vi "ReadSeq_Analyze.vi"(6 "RotateAngle":string, 7 "Color":u32(colorbox)=16711680, 8 "error in (no error)":errorcluster, 9 "Cam Index":i32, 10 "script path":string, 11 "coordinate space":bool) -> (0 "error out":errorcluster, 1 "data string":string, 2 "Description":string, 3 "VarName":string)   [LabVIEW 2015]
panel:
  out "x-y":u32
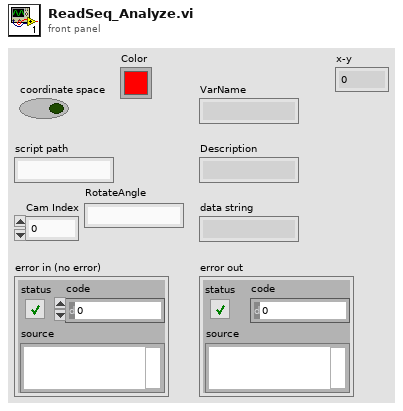
[diagram p1: front panel]
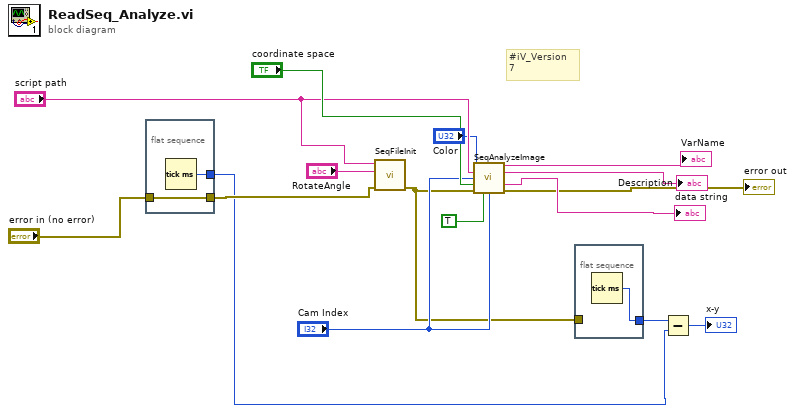
[diagram p0: block diagram]
diagram:
  # "#iV_Version\n7"
  n1 = flat-sequence {
    tunnel: "error in (no error)" -> [w18]
    tunnel: [w18] -> w6
    tunnel: [w17] -> w3
    frame #0 {
      n2 = Tick Count (ms)() -> (millisecond timer value=w17:u32)
    }
  }
  n3 = call "SeqFileInit.vi"("error in (no error)"=w6, "RotateAngle"="RotateAngle", "script path"="script path") -> ("error out"=w5:errorcluster)  [unwired: 7 in, 1 out]
  n4 = call "SeqAnalyzeImage.vi"("Color"="Color", "Script Path"="script path", "Index"="Cam Index", "coordinate space"="coordinate space", "error in"=w5, "CreatDllImage"=TRUE, "Cam Index"="Cam Index") -> ("VarName"=→"VarName":string, "Description"=→"Description":string, "data string"=→"data string":string, "error out"=→"error out":errorcluster)  [unwired: 3 in, 2 out]
  n5 = flat-sequence {
    tunnel: w5 -> [_]
    tunnel: [w19] -> w4
    frame #0 {
      n6 = Tick Count (ms)() -> (millisecond timer value=w19:u32)
    }
  }
  n7 = Subtract(x=w4, y=w3) -> (x-y=→"x-y":u32)
